vi "FT10_Log Update Bipolar Log.vi"(10 "Bipolar Activate":T1, 11 "Message Handling Cluster in":T2) -> (3 "Message Handling Cluster out":T2)   [LabVIEW 2015]
doc: "Update \"Log Activation Settings Cluster\" with the Bipolas Port and Mode."
uses:
  Controls/Control_Message Handling Cluster.ctl
  Controls/Control_M4X Connection.ctl
  Controls/Control_PXI-7854R FPGA Reference.ctl
  Controls/Control_Config Cluster.ctl
  Controls/Control_Config Unitherm Port.ctl
  Controls/Control_Config Simulate Values.ctl
  Controls/Control_Config Fornax Connect Attempts.ctl
  Controls/Control_Log Queue.ctl
  Controls/Control_Log Cluster.ctl
  Controls/Control_Log Time.ctl
  Controls/Control_Log Waveform Cluster - Current.ctl
  Controls/Control_Log Analysis Cluster - Current.ctl
  Controls/Control_Log Activation Settings Cluster.ctl
  Controls/Control_Log Unitherm Load.ctl
  Controls/Control_Log Port.ctl
  Controls/Control_Log Mode.ctl
  Controls/Control_Log Power Level.ctl
  Controls/Control_Log Waveform Cluster - Diff Voltage.ctl
  Controls/Control_Log Analysis Cluster - Diff Voltage.ctl
  Controls/Control_Log Flag.ctl
  Controls/Control_Log Port Mode Cluster.ctl
  Controls/Control_Fornax Mono1 Cut Enum.ctl
  Controls/Control_Fornax Mono2 Cut Enum.ctl
  Controls/Control_Fornax Mono1 Coag Enum.ctl
  Controls/Control_Fornax Mono2 Coag Enum.ctl
  Controls/Control_Fornax Bipolar Enum.ctl
  Controls/Control_Indicator Cluster.ctl
  Controls/Control_Log Power Level Cluster.ctl
  Controls/Control_Log Mono1 Cut Power.ctl
  Controls/Control_Log Mono1 Coag Power.ctl
  Controls/Control_Log Mono2 Cut Power.ctl
  Controls/Control_Log Mono2 Coag Power.ctl
  Controls/Control_Log Bipolar Power.ctl
  Controls/Control_Fornax Bipolar Activate Port Bool.ctl
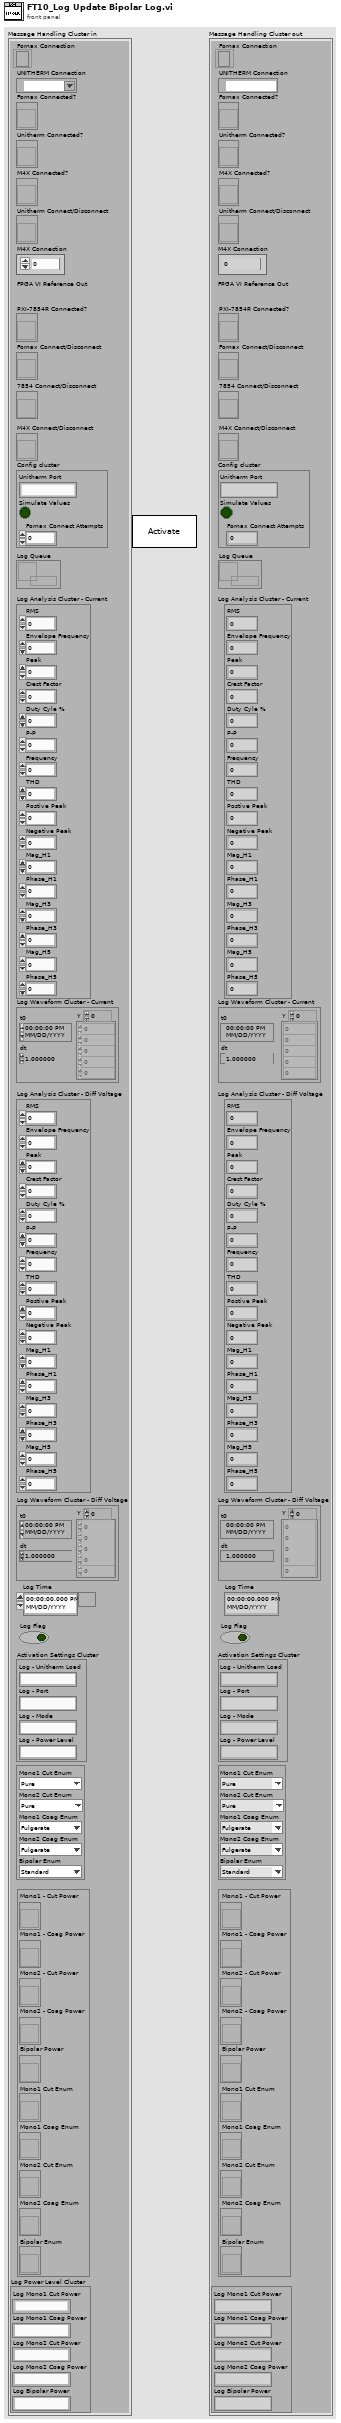
[diagram p1: front panel]
types:
  T1 = typedef "Control_Fornax Bipolar Activate Port Bool.ctl" = bool
  T2 = typedef "Control_Message Handling Cluster.ctl" = cluster{"Fornax Connected?":refnum<vi>, "Unitherm Connected?":refnum<vi>, "M4X Connected?":refnum<vi>, "Unitherm Connect/Disconnect":refnum<vi>, "Fornax Connection":refnum<k5>, "UNITHERM Connection":refnum<visa-resource-name>, "M4X Connection":T3, "FPGA VI Reference Out":T4, "PXI-7854R Connected?":refnum<vi>, "Fornax Connect/Disconnect":refnum<vi>, "7854 Connect/Disconnect":refnum<vi>, "M4X Connect/Disconnect":refnum<vi>, "Config cluster":T5, "Log Queue":T9, "Log Analysis Cluster - Current":T10, "Log Waveform Cluster - Current":T11, "Log Time":T12, "Log Flag":T13, "Log - Activation Settings Cluster":T14, "Log - Port Mode Cluster":T19, "Log Analysis Cluster - Diff Voltage":T25, "Log Waveform Cluster - Diff Voltage":T26, "Indicator Cluster":T27, "Log Power Level Cluster":T28}
  T3 = typedef "Control_M4X Connection.ctl" = u32
  T4 = typedef "Control_PXI-7854R FPGA Reference.ctl" = refnum<k20>
  T5 = typedef "Control_Config Cluster.ctl" = cluster{"Unitherm Port":T6, "Simulate Values":T7, "Fornax Connect Attempts":T8}
  T6 = typedef "Control_Config Unitherm Port.ctl" = string
  T7 = typedef "Control_Config Simulate Values.ctl" = bool
  T8 = typedef "Control_Config Fornax Connect Attempts.ctl" = i32
  T9 = typedef "Control_Log Queue.ctl" = refnum<queue>
  T10 = typedef "Control_Log Analysis Cluster - Current.ctl" = cluster{"RMS":dbl, "Envelope Frequency":dbl, "Peak":dbl, "Crest Factor":dbl, "Duty Cyle %":dbl, "P-P":dbl, "Frequency":dbl, "THD":dbl, "Postive Peak":dbl, "Negative Peak":dbl, "Mag_H1":dbl, "Phase_H1":dbl, "Mag_H3":dbl, "Phase_H3":dbl, "Mag_H5":dbl, "Phase_H5":dbl}
  T11 = typedef "Control_Log Waveform Cluster - Current.ctl" = waveform(dbl)
  T12 = typedef "Control_Log Time.ctl" = timestamp
  T13 = typedef "Control_Log Flag.ctl" = bool
  T14 = typedef "Control_Log Activation Settings Cluster.ctl" = cluster{"Log - Unitherm Load":T15, "Log - Port":T16, "Log - Mode":T17, "Log - Power Level":T18}
  T15 = typedef "Control_Log Unitherm Load.ctl" = string
  T16 = typedef "Control_Log Port.ctl" = string
  T17 = typedef "Control_Log Mode.ctl" = string
  T18 = typedef "Control_Log Power Level.ctl" = string
  T19 = typedef "Control_Log Port Mode Cluster.ctl" = cluster{"Mono1 Cut Enum":T20, "Mono2 Cut Enum":T21, "Mono1 Coag Enum":T22, "Mono2 Coag Enum":T23, "Bipolar Enum":T24}
  T20 = typedef "Control_Fornax Mono1 Cut Enum.ctl" = enum16{"Pure", "Blend"}
  T21 = typedef "Control_Fornax Mono2 Cut Enum.ctl" = enum16{"Pure", "Blend"}
  T22 = typedef "Control_Fornax Mono1 Coag Enum.ctl" = enum16{"Fulgerate", "Spray"}
  T23 = typedef "Control_Fornax Mono2 Coag Enum.ctl" = enum16{"Fulgerate", "Spray"}
  T24 = typedef "Control_Fornax Bipolar Enum.ctl" = enum16{"Standard", "Macro", "Precision"}
  T25 = typedef "Control_Log Analysis Cluster - Diff Voltage.ctl" = cluster{"RMS":dbl, "Envelope Frequency":dbl, "Peak":dbl, "Crest Factor":dbl, "Duty Cyle %":dbl, "P-P":dbl, "Frequency":dbl, "THD":dbl, "Postive Peak":dbl, "Negative Peak":dbl, "Mag_H1":dbl, "Phase_H1":dbl, "Mag_H3":dbl, "Phase_H3":dbl, "Mag_H5":dbl, "Phase_H5":dbl}
  T26 = typedef "Control_Log Waveform Cluster - Diff Voltage.ctl" = waveform(dbl)
  T27 = typedef "Control_Indicator Cluster.ctl" = cluster{"Mono1 - Cut Power":refnum<vi>, "Mono1 - Coag Power":refnum<vi>, "Mono2 - Cut Power":refnum<vi>, "Mono2 - Coag Power":refnum<vi>, "Bipolar Power":refnum<vi>, "Mono1 Cut Enum":refnum<vi>, "Mono1 Coag Enum":refnum<vi>, "Mono2 Cut Enum":refnum<vi>, "Mono2 Coag Enum":refnum<vi>, "Bipolar Enum":refnum<vi>}
  T28 = typedef "Control_Log Power Level Cluster.ctl" = cluster{"Log Mono1 Cut Power":T29, "Log Mono1 Coag Power":T30, "Log Mono2 Cut Power":T31, "Log Mono2 Coag Power":T32, "Log Bipolar Power":T33}
  T29 = typedef "Control_Log Mono1 Cut Power.ctl" = string
  T30 = typedef "Control_Log Mono1 Coag Power.ctl" = string
  T31 = typedef "Control_Log Mono2 Cut Power.ctl" = string
  T32 = typedef "Control_Log Mono2 Coag Power.ctl" = string
  T33 = typedef "Control_Log Bipolar Power.ctl" = string
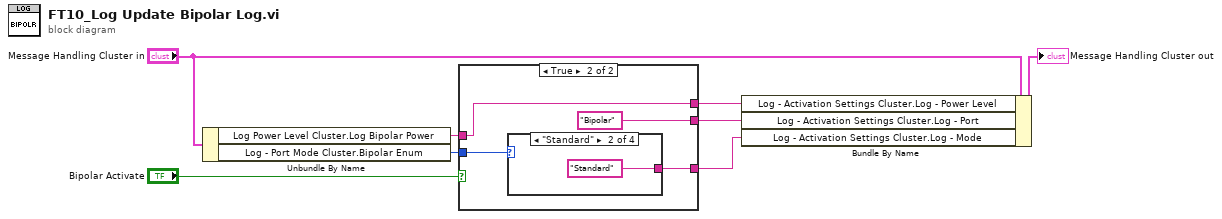
[diagram p0: block diagram]
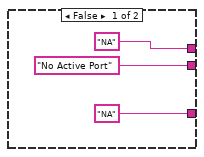
[diagram p2: hidden frame]
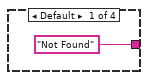
[diagram p3: hidden frame]
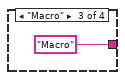
[diagram p4: hidden frame]
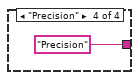
[diagram p5: hidden frame]
diagram:
  n1 = Unbundle By Name("Message Handling Cluster in") -> ("Log Power Level Cluster.Log Bipolar Power"=w1:T33, "Log - Port Mode Cluster.Bipolar Enum"=w5:T24)
  n2 = case shown="True" "Bipolar Activate" {
    tunnel: w5 -> [_ w15]
    tunnel: [T16 "No Active Port" ("Log - Activation Settings Cluster.Log - Port") T16 "Bipolar" ("Log - Activation Settings Cluster.Log - Port")] -> w6
    tunnel: [T17 "NA" ("Log - Activation Settings Cluster.Log - Mode") w13] -> w7
    tunnel: [T18 "NA" ("Log - Activation Settings Cluster.Log - Power Level") w12] -> w2
    tunnel: w1 -> [_ w12]
    frame False {
    }
    frame True {
      n3 = case shown="\"Standard\"" w15 {
        tunnel: [T17 "Not Found" ("Log - Activation Settings Cluster.Log - Mode") T17 "Standard" ("Log - Activation Settings Cluster.Log - Mode") T17 "Macro" ("Log - Activation Settings Cluster.Log - Mode") T17 "Precision" ("Log - Activation Settings Cluster.Log - Mode")] -> w13
        frame Default {
        }
        frame "Standard" {
        }
        frame "Macro" {
        }
        frame "Precision" {
        }
      }
    }
  }
  n4 = Bundle By Name(cluster="Message Handling Cluster in", "Log - Activation Settings Cluster.Log - Power Level"=w2, "Log - Activation Settings Cluster.Log - Port"=w6, "Log - Activation Settings Cluster.Log - Mode"=w7) -> (→"Message Handling Cluster out":T2)
